vi "随机数出数.vi"(6 "信号值原始值":dbl, 7 "公式":cluster{"X^2":dbl, "X":dbl, "B":dbl}, 8 "启用":bool, 9 "采样值":dbl[](array[numeric]), 10 "参数输入":T1={"采样模式"=enum."自动采样", "采样点数"=3, "变异系数设定值"=0.1, "重新取值百分比"=0.5, "偏差模式"=enum."相对偏差", "相对偏差百分比"=0.0, "绝对偏差值"=0.0}, 11 "监测值原始值":dbl) -> (1 "采样值输出":dbl[](array[numeric]), 2 "参数输出":cluster{"mean":dbl, "变异系数":dbl, "随机数？":bool} {"mean" format="%0.2f"}, 3 "取值输出":dbl, 4 "信号值":dbl)   [LabVIEW 2016, in "random number.lvlib"]
uses:
  random number.lvlib
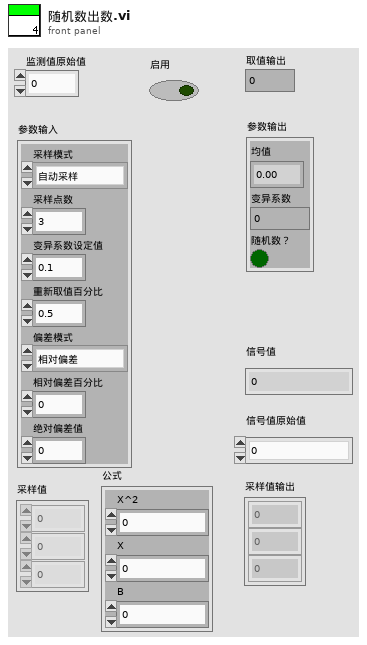
[diagram p1: front panel]
types:
  T1 = cluster{"采样模式":enum16{"自动采样", "手动采样"}, "采样点数":i32, "变异系数设定值":dbl, "重新取值百分比":dbl, "偏差模式":enum16{"相对偏差", "绝对偏差"}, "相对偏差百分比":dbl, "绝对偏差值":dbl}
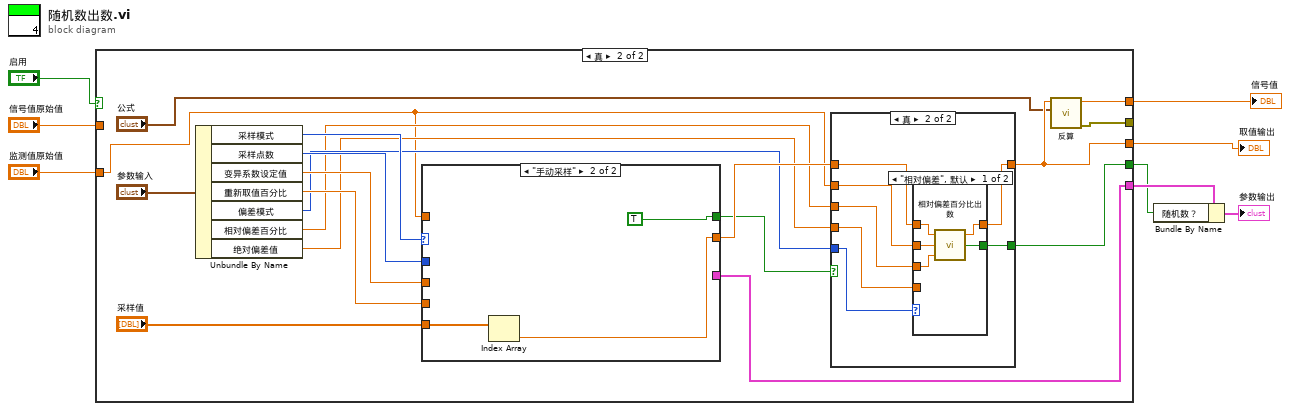
[diagram p0: block diagram]
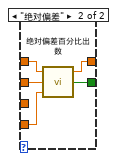
[diagram p4: hidden frame]
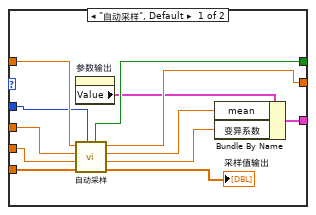
[diagram p5: hidden frame]
diagram:
  n1 = case shown="真" "启用" {
    tunnel: "监测值原始值" -> [w10 w13]
    tunnel: [w10 w17] -> w7
    tunnel: [_ w15] -> _
    tunnel: "信号值原始值" -> [w9 _]
    tunnel: [w9 w14] -> w4
    tunnel: [_ w12] -> w1
    tunnel: [_ w11] -> w3
    frame False {
    }
    frame True {
      n2 = Unbundle By Name("参数输入") -> ("采样模式"=w25:enum16{"自动采样", "手动采样"}, "采样点数"=w24:i32, "变异系数设定值"=w23:dbl, "重新取值百分比"=w22:dbl, "偏差模式"=w21:enum16{"相对偏差", "绝对偏差"}, "相对偏差百分比"=w20:dbl, "绝对偏差值"=w19:dbl)
      n3 = case shown="\"手动采样\"" w25 {
        tunnel: [w58 w59] -> w28
        tunnel: w13 -> [w57 _]
        tunnel: [w56 TRUE ("采样OK")] -> w27
        tunnel: w24 -> [w55 _]
        tunnel: w23 -> [w54 _]
        tunnel: w22 -> [w53 _]
        tunnel: "采样值" -> [w49 w60]
        tunnel: [w47 _] -> w11
        frame "自动采样", Default {
          n4 = property on="参数输出" class="Clust (严格)"() -> ("Value"=w52:cluster{"mean":dbl, "变异系数":dbl, "随机数？":bool})  [unwired: 2 in, 2 out]
          n5 = call "自动采样.vi"("采样点数"=w55, "采样值"=w49, "重新取值百分比"=w53, "变异系数设定值"=w54, "原始值"=w57) -> ("采样值输出"=→"采样值输出":dbl[], "变异系数"=w50:dbl, "mean"=w51:dbl, "取值输出"=w58:dbl, "采样OK"=w56:bool)  [unwired: 2 in]
          n6 = Bundle By Name(cluster=w52, "mean"=w51, "变异系数"=w50) -> (w47:cluster{"mean":dbl, "变异系数":dbl, "随机数？":bool})
        }
        frame "手动采样" {
          n7 = Index Array(array=w60) -> (element=w59:dbl)  [unwired: 1 in]
        }
      }
      n8 = case shown="真" w27 {
        tunnel: w28 -> [w29 w36]
        tunnel: [w29 w35] -> w17
        tunnel: w21 -> [_ w34]
        tunnel: w20 -> [_ w33]
        tunnel: w19 -> [_ w32]
        tunnel: w13 -> [_ w31]
        tunnel: [_ w30] -> w12
        frame False {
        }
        frame True {
          n9 = case shown="\"相对偏差\", 默认" w34 {
            tunnel: w36 -> [w41 w46]
            tunnel: [w40 w45] -> w35
            tunnel: w33 -> [w39 _]
            tunnel: w32 -> [_ w44]
            tunnel: w31 -> [w38 w42]
            tunnel: [w37 w43] -> w30
            frame "相对偏差", Default {
              n10 = call "相对偏差百分比出数.vi"("基准值"=w41, "原始值"=w38, "相对偏差百分比"=w39) -> ("取值输出"=w40:dbl, "随机数？"=w37:bool)  [unwired: 5 in]
            }
            frame "绝对偏差" {
              n11 = call "绝对偏差百分比出数.vi"("基准值"=w46, "原始值"=w42, "绝对偏差值"=w44) -> ("取值输出"=w45:dbl, "随机值？"=w43:bool)  [unwired: 5 in]
            }
          }
        }
      }
      n12 = call "反算.vi"("公式"="公式", "监测值"=w17) -> ("error out"=w15:errorcluster, "信号值"=w14:dbl)  [unwired: 8 in]
    }
  }
  "取值输出" <- w7
  "信号值" <- w4
  n13 = Bundle By Name(cluster=w3, "随机数？"=w1) -> (→"参数输出":cluster{"mean":dbl, "变异系数":dbl, "随机数？":bool})
